vi "Subvi AO trigger pockels.vi"(8 "SecondaryDelay_tick":u32, 9 "MainDelay_tick":u32, 11 "Trigger":bool) -> (1 "IteratorDirection":bool, 3 "Stop":bool, 4 "Framecount":i16)   [LabVIEW 2017]
uses:
  GV trigger external AODO.vi
  GV Nframes.vi
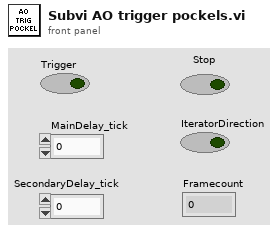
[diagram p1: front panel]
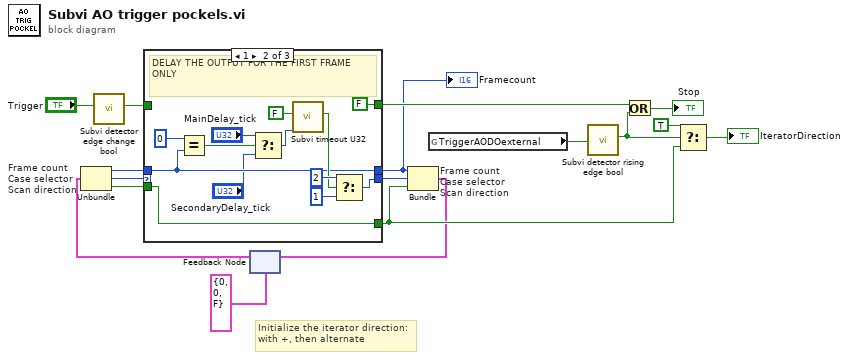
[diagram p0: block diagram]
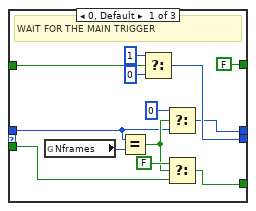
[diagram p2: hidden frame]
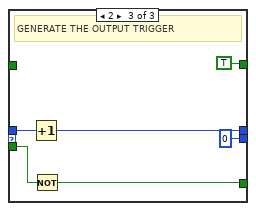
[diagram p3: hidden frame]
diagram:
  # "Initialize the iterator direction:\nwith +, then alternate"
  n1 = call "Subvi detector edge change bool.vi"("Input"="Trigger") -> ("Output"=w8:bool)  [unwired: 8 in]
  n2 = feedback #1(cluster{i16, "f":u8, bool} {0, "f"=0, FALSE}) -> (w6:cluster{i16, "f":u8, bool})
  n3 = Unbundle "Frame count\nCase selector\nScan direction"(w6) -> (w5:i16, "f"=w3:u8, w4:bool)
  n4 = case shown="1" w3 {
    tunnel: [w30 w41 u8 0 ("f")] -> w15
    tunnel: [FALSE FALSE TRUE] -> w11
    tunnel: [w19 w39 w47] -> w12
    tunnel: w8 -> [w26 _ _]
    tunnel: [w23 w33 w44] -> w1
    tunnel: w4 -> [w22 w39 w46]
    tunnel: w5 -> [w18 w33 w45]
    frame 0, Default {
      # "WAIT FOR THE MAIN TRIGGER"
      n5 = global read "GV Nframes.vi" "Nframes"() -> (w25:i16)
      n6 = Equal?(x=w18, y=w25) -> (x = y?=w20:bool)
      n7 = Select(t=u8 1, s=w26, f=u8 0) -> (s? t:f=w30:u8)
      n8 = Select(t=i16 0, s=w20, f=w18) -> (s? t:f=w23:i16)
      n9 = Select(t=FALSE, s=w20, f=w22) -> (s? t:f=w19:bool)
    }
    frame 1 {
      # "DELAY THE OUTPUT FOR THE FIRST FRAME ONLY"
      n10 = Equal?(x=i16 0, y=w33) -> (x = y?=w36:bool)
      n11 = Select(t="MainDelay_tick", s=w36, f="SecondaryDelay_tick") -> (s? t:f=w35:u32)
      n12 = call "Subvi timeout U32.vi"("Timeout_tick"=w35, "Input"=FALSE) -> ("Timeout"=w37:bool)  [unwired: 9 in]
      n13 = Select(t=u8 2, s=w37, f=u8 1) -> (s? t:f=w41:u8)
    }
    frame 2 {
      # "GENERATE THE OUTPUT TRIGGER"
      n14 = Increment(x=w45) -> (x+1=w44:i16)
      n15 = Not(x=w46) -> (.not. x?=w47:bool)
    }
  }
  "Framecount" <- w1
  n16 = Bundle "Frame count\nCase selector\nScan direction"(w1, "f"=w15, "t"=w12) -> (w7:cluster{i16, "f":u8, "t":bool})  [unwired: 1 in]
  n17 = feedback-in #1(w7) -> ()
  n18 = global read "GV trigger external AODO.vi" "TriggerAODOexternal"() -> (w17:bool)
  n19 = call "Subvi detector rising edge bool.vi"("Input"=w17) -> ("Output"=w10:bool)  [unwired: 10 in]
  n20 = Or(x=w11, y=w10) -> (x .or. y?=→"Stop":bool)
  n21 = Select(t=TRUE, s=w10, f=w12) -> (s? t:f=→"IteratorDirection":bool)
